vi "Add Rx UDP information.vi"(8 "error in":errorcluster, 11 "incoming ref":T1 format="%.0x") -> (0 "error out":errorcluster, 3 "incoming ref out":T1 format="%.0x")   [LabVIEW 2020, in "AIM ARINC 664 Scripting.lvlib"]
doc: "Add a Rx UDP page."
uses:
  AIM ARINC 664 Scripting.lvlib
  <vilib>/NI VeriStand/Custom Device API/Custom Device Item Ref.ctl
  <vilib>/NI VeriStand/Custom Device API/Custom Device Channel.ctl
  <vilib>/NI VeriStand/Custom Device API/Custom Device Channel Type.ctl
  Constants.vi
  <vilib>/NI VeriStand/Custom Device API/Custom Device API.lvlib
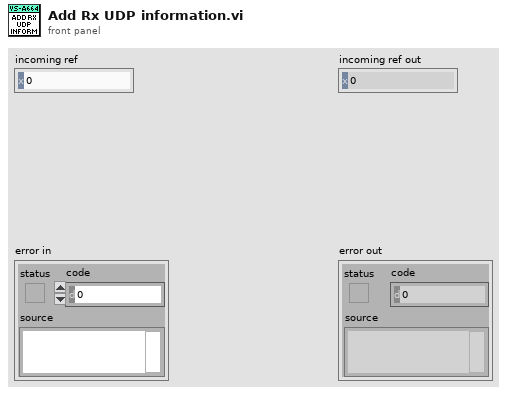
[diagram p1: front panel]
types:
  T1 = typedef "Custom Device API.lvlib/Custom Device Item Ref.ctl" = u64
  T2 = typedef "Custom Device API.lvlib/Custom Device Channel.ctl" = cluster{"Type":T3, "Units":string, "Default Value":dbl, "Faultable":bool, "Scalable":bool}
  T3 = typedef "Custom Device API.lvlib/Custom Device Channel Type.ctl" = enum16{"Input", "Output"}
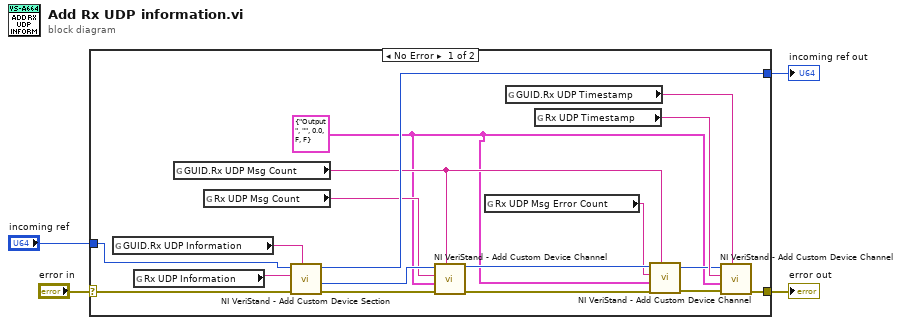
[diagram p0: block diagram]
diagram:
  n1 = case shown="No Error" "error in" {
    selector: "error in" -> [w20 w24]
    tunnel: "incoming ref" -> [w21 w23]
    tunnel: [w22 w24] -> w3
    tunnel: [w19 w23] -> w2
    frame No Error {
      w5 = T2 {"Type"=enum."Output", "Units"="", "Default Value"=0.0, "Faultable"=FALSE, "Scalable"=FALSE} ("Channel")
      n2 = global read "Constants.vi" "GUID.Rx UDP Information"() -> (w13:string)
      n3 = global read "Constants.vi" "Rx UDP Information"() -> (w12:string)
      n4 = global read "Constants.vi" "GUID.Rx UDP Msg Count"() -> (w11:string)
      n5 = global read "Constants.vi" "Rx UDP Msg Count"() -> (w15:string)
      n6 = call <vilib>:"NI VeriStand - Add Custom Device Section.vi"("GUID (Default Section)"=w13, "error in (no error)"=w20, "Section Name"=w12, "Parent Ref in"=w21) -> ("error out"=w17:errorcluster, "Section Ptr"=w18:T1, "Parent Ref out"=w19:T1)  [unwired: 4 in, 1 out]
      n7 = call <vilib>:"NI VeriStand - Add Custom Device Channel.vi"("GUID (Default Channel)"=w11, "error in (no error)"=w17, "Channel"=w5, "Channel Name"=w15, "Parent Ref in"=w18) -> ("error out"=w9:errorcluster, "Parent Ref out"=w10:T1)  [unwired: 3 in, 2 out]
      n8 = global read "Constants.vi" "Rx UDP Msg Error Count"() -> (w6:string)
      n9 = global read "Constants.vi" "GUID.Rx UDP Timestamp"() -> (w16:string)
      n10 = global read "Constants.vi" "Rx UDP Timestamp"() -> (w14:string)
      n11 = call <vilib>:"NI VeriStand - Add Custom Device Channel.vi"("GUID (Default Channel)"=w11, "error in (no error)"=w9, "Channel"=w5, "Channel Name"=w6, "Parent Ref in"=w10) -> ("error out"=w8:errorcluster, "Parent Ref out"=w7:T1)  [unwired: 3 in, 2 out]
      n12 = call <vilib>:"NI VeriStand - Add Custom Device Channel.vi"("GUID (Default Channel)"=w16, "error in (no error)"=w8, "Channel"=w5, "Channel Name"=w14, "Parent Ref in"=w7) -> ("error out"=w22:errorcluster)  [unwired: 3 in, 3 out]
    }
    frame Error {
    }
  }
  "error out" <- w3
  "incoming ref out" <- w2
